vi "MKS_RELAYS (SubVI).vi"(8 "error in (no error)":errorcluster, 11 "Cluster in":T1 caption="Cluster 2" {"parity (0:none)" items=["None", "Odd", "Even", "Mark", "Space"]; "BAUDE RATE" items=["38400"=38400, "19200"=19200, "9600"=9600, "4800"=4800]}) -> (0 "error out":errorcluster, 3 "x != 0?":bool[](array[boolean]))   [LabVIEW 2020]
uses:
  INITIALIZATION.ctl
  <vilib>/Instr/_visa.llb/VISA Configure Serial Port (Instr).vi
  <instrlib>/PV ActiveLine/PV ActiveLine.lvlib
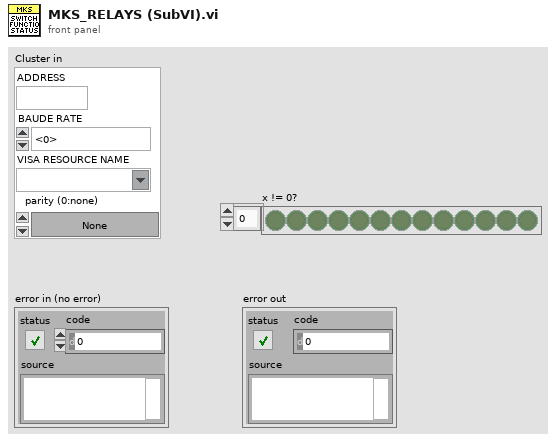
[diagram p1: front panel]
types:
  T1 = typedef "INITIALIZATION.ctl" = cluster{"ADDRESS":string, "BAUDE RATE":u32, "VISA RESOURCE NAME":refnum<visa-resource-name>, "parity (0:none)":u16}
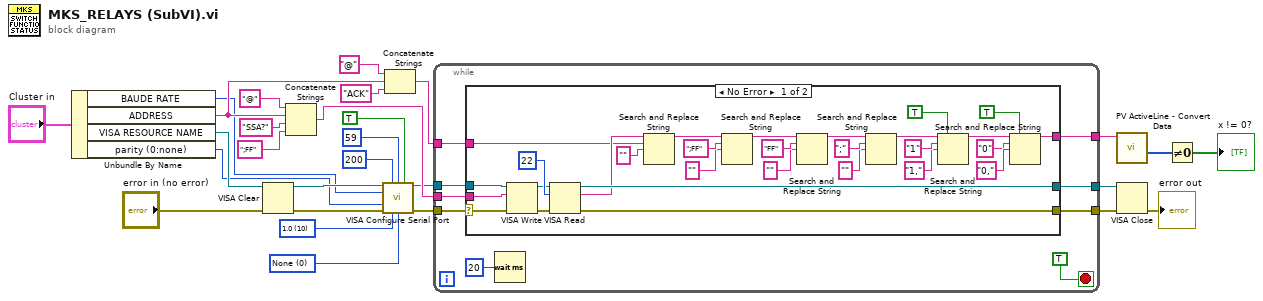
[diagram p0: block diagram]
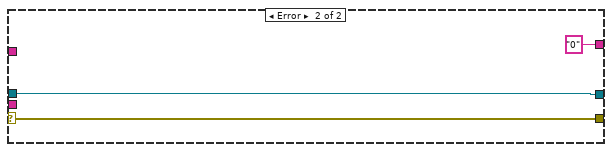
[diagram p2: hidden frame]
diagram:
  w15 = u16 0 items=["None", "XON/XOFF", "RTS/CTS", "XON/XOFF & RTS/CTS", "DTR/DSR", "XON/XOFF & DTR/DSR"] ("flow control (0:none)")
  w9 = u16 10 items=["1.0"=10, "1.5"=15, "2.0"=20] ("stop bits (10: 1 bit)")
  n1 = Unbundle By Name("Cluster in") -> ("BAUDE RATE"=w10:u32, "ADDRESS"=w17:string, "VISA RESOURCE NAME"=w27:refnum<visa-resource-name>, "parity (0:none)"=w16:u16)
  n2 = VISA Clear(VISA resource name=w27, error in (no error)="error in (no error)") -> (VISA resource name out=w26:refnum<visa-resource-name>, error out=w28:errorcluster)
  n3 = Concatenate Strings("@" ("string"), w17, "SSA?" ("string"), ";FF" ("string")) -> (w22:string)
  n4 = call-poly "VISA Configure Serial Port"("VISA resource name"=w26, "timeout (10sec)"=u32 200, "termination char\n(0xA = '\\n' = LF)"=u8 59, "Enable Termination\nChar (T)"=TRUE ("Enable Termination\nChar (T)"), "baud rate (9600)"=w10, "parity (0:none)"=w16, "error in (no error)"=w28, "stop bits (10: 1 bit)"=w9, "flow control (0:none)"=w15) -> ("VISA resource name out"=w13:refnum<visa-resource-name>, "error out"=w14:errorcluster)  [unwired: 5 in]
  n5 = Concatenate Strings("@" ("search string"), w17, "ACK" ("string")) -> (w25:string)
  n6 = while {
    tunnel: w14 -> [w29]
    tunnel: [w36] -> w18
    tunnel: w13 -> [w37]
    tunnel: [w35] -> w5
    tunnel: w22 -> [w32]
    tunnel: w25 -> [w31]
    tunnel: [w30] -> w4
    stop <- TRUE stop-if-true
    n7 = case shown="No Error" w29 {
      selector: w29 -> [w38 w67]
      tunnel: w37 -> [w66 w68]
      tunnel: [w65 w67] -> w36
      tunnel: [w64 w68] -> w35
      tunnel: w32 -> [w57 _]
      tunnel: w31 -> [w56 _]
      tunnel: [w41 "0" ("result string")] -> w30
      frame No Error {
        n8 = VISA Write(VISA resource name=w66, write buffer=w57, error in (no error)=w38) -> (VISA resource name out=w49:refnum<visa-resource-name>, error out=w48:errorcluster)  [unwired: 1 out]
        n9 = VISA Read(VISA resource name=w49, byte count=u32 22, error in (no error)=w48) -> (VISA resource name out=w64:refnum<visa-resource-name>, read buffer=w62:string, error out=w65:errorcluster)  [unwired: 1 out]
        n10 = Search and Replace String(input string=w62, search string=w56, replace string="" ("replace string (\"\")")) -> (result string=w60:string)  [unwired: 5 in, 3 out]
        n11 = Search and Replace String(input string=w60, search string=";FF", replace string="" ("replace string (\"\")")) -> (result string=w52:string)  [unwired: 5 in, 3 out]
        n12 = Search and Replace String(input string=w52, search string="FF", replace string="" ("replace string (\"\")")) -> (result string=w51:string)  [unwired: 5 in, 3 out]
        n13 = Search and Replace String(input string=w51, search string=";", replace string="" ("replace string (\"\")")) -> (result string=w47:string)  [unwired: 5 in, 3 out]
        n14 = Search and Replace String(replace all?=TRUE ("replace all? (F)"), input string=w47, search string="1", replace string="1," ("replace string (\"\")")) -> (result string=w43:string)  [unwired: 4 in, 3 out]
        n15 = Search and Replace String(replace all?=TRUE ("replace all? (F)"), input string=w43, search string="0", replace string="0," ("replace string (\"\")")) -> (result string=w41:string)  [unwired: 4 in, 3 out]
      }
      frame Error {
      }
    }
    n16 = Wait (ms)(milliseconds to wait=u32 20) -> ()  [unwired: 1 out]
  }
  n17 = call <instrlib>:"PV ActiveLine - Convert Data.vi"("String in"=w4) -> ("Integer Out"=w2:i32[])  [unwired: 7 in, 3 out]
  n18 = VISA Close(VISA resource name=w5, error in (no error)=w18) -> (error out=→"error out":errorcluster)
  n19 = Not Equal To 0?(x=w2) -> (x != 0?=→"x != 0?":bool[])
